vi "菜单-下载.vi"(8 "error in (no error)":errorcluster caption="错误输入（无错误）", 11 "程序响应 输入":refnum<class "程序响应.lvclass">) -> (0 "error out":errorcluster caption="错误输出", 3 "程序响应 输出":refnum<class "程序响应.lvclass">)   [LabVIEW 2020, in "程序响应.lvlib" / "程序响应.lvclass"]
uses:
  D:/SuperPython-master/ScintillaNET.dll
  ScintillaNET.dll
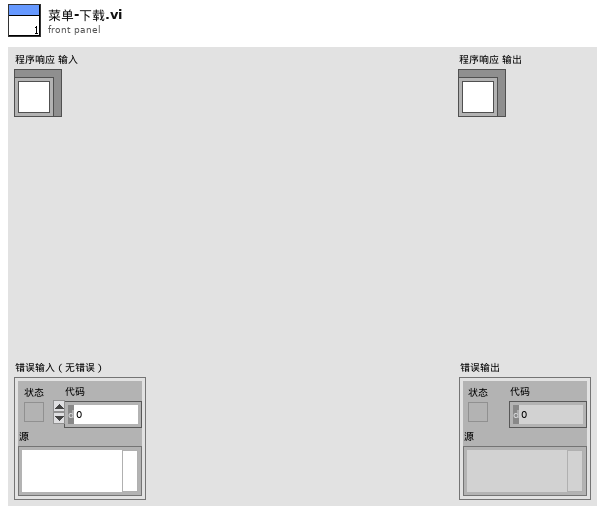
[diagram p1: front panel]
types:
  T1 = enum16{"open", "replace", "create", "open or create", "replace or create", "replace or create with confirmation"}
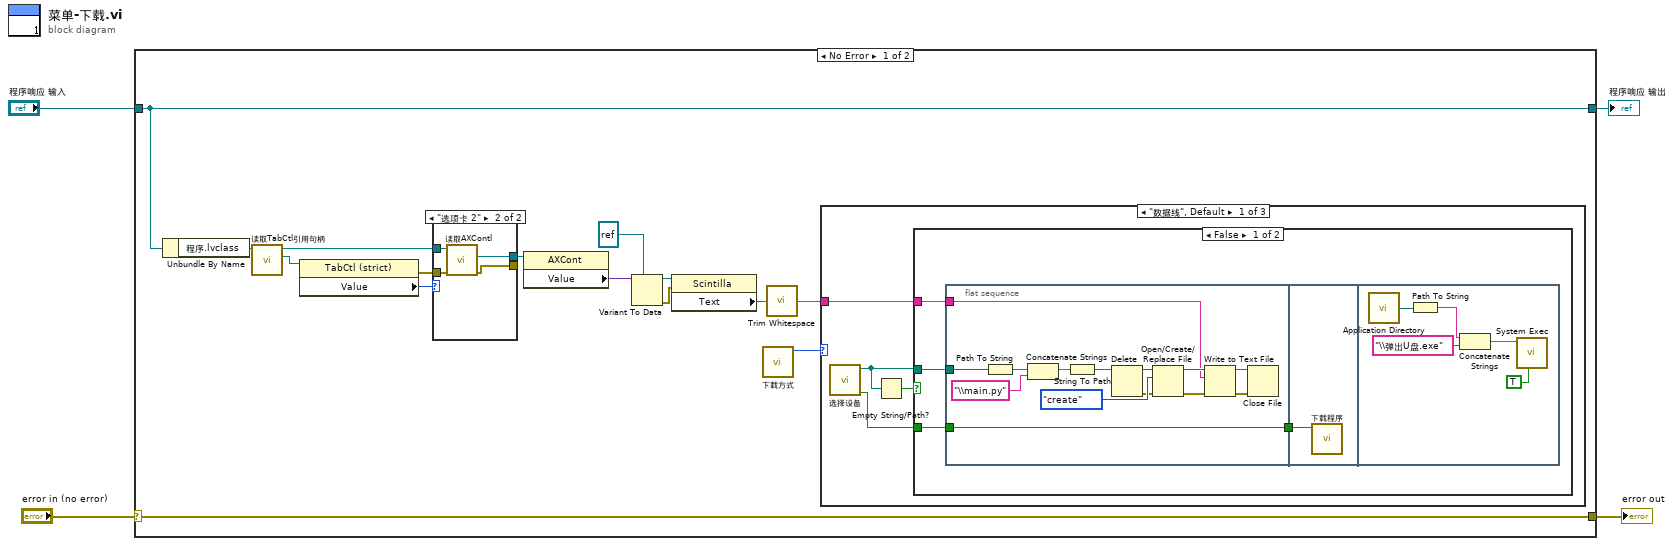
[diagram p0: block diagram]
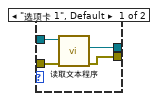
[diagram p2: hidden frame]
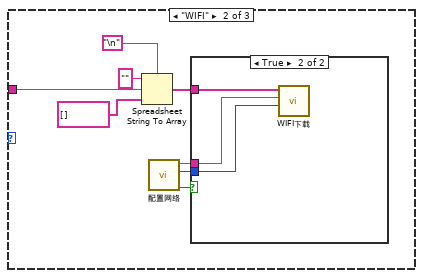
[diagram p4: hidden frame]
diagram:
  n1 = case shown="No Error" "error in (no error)" {
    selector: "error in (no error)" -> [w19 w68]
    tunnel: [w19 w68] -> w3
    tunnel: [w18 w67] -> w1
    tunnel: "程序响应 输入" -> [w18 w67]
    frame No Error {
      n2 = Unbundle By Name(w18) -> ("程序.lvclass"=w5:refnum<class "程序.lvclass">)
      n3 = call-dynamic "读取TabCtl引用句柄.vi"("程序输入"=w5) -> ("TabCtl引用句柄"=w10:refnum<vi>, "程序输出"=w7:refnum<class "程序.lvclass">)  [unwired: 8 in, 1 out]
      n4 = property class="TabCtl (strict)"(reference=w10) -> (error out=w8:errorcluster, "Value"=w9:enum32{"选项卡 1", "选项卡 2"})  [unwired: 1 in, 1 out]
      n5 = case shown="\"选项卡 2\"" w9 {
        tunnel: [w23 w24] -> w6
        tunnel: [w21 w25] -> _
        tunnel: w7 -> [w22 w27]
        tunnel: w8 -> [w20 w26]
        frame "选项卡 1", Default {
          n6 = call-dynamic "读取文本程序.vi"("error in (no error)"=w20, "程序输入"=w22) -> ("error out"=w21:errorcluster, "文本程序"=w23:refnum<vi>)  [unwired: 7 in, 1 out]
        }
        frame "选项卡 2" {
          n7 = call-dynamic "读取AXContl.vi"("error in (no error)"=w26, "程序输入"=w27) -> ("error out"=w25:errorcluster, "AXContl"=w24:refnum<vi>)  [unwired: 7 in, 1 out]
        }
      }
      n8 = property class="AXCont"(reference=w6) -> ("Value"=w12:variant)  [unwired: 1 in, 2 out]
      n9 = Variant To Data(type=refnum<k24> refnum ("文本编辑"), Variant=w12) -> (data=w13:refnum<k24>, error out=w14:errorcluster)  [unwired: 1 in]
      n10 = property class="Scintilla"(reference=w13, error in=w14) -> ("Text"=w11:string)  [unwired: 2 out]
      n11 = call "下载方式.vi"() -> ("下载方式"=w17:enum32{"数据线", "WIFI", "取消"})  [unwired: 11 in]
      n12 = call <vilib>:"Trim Whitespace.vi"("string"=w11) -> ("trimmed string"=w16:string)  [unwired: 1 in]
      n13 = case shown="\"数据线\", Default" w17 {
        tunnel: w16 -> [w31 w63 _]
        frame "数据线", Default {
          n14 = call "选择设备.vi"() -> ("boot?"=w28:bool, "路径"=w30:path)  [unwired: 10 in]
          n15 = Empty String/Path?(string/path=w30) -> (empty?=w29:bool)
          n16 = case shown="False" w29 {
            tunnel: w30 -> [w34 _]
            tunnel: w31 -> [w35 _]
            tunnel: w28 -> [w33 _]
            frame False {
              n17 = flat-sequence {
                tunnel: w35 -> [w44]
                tunnel: w34 -> [w43]
                tunnel: w33 -> [w36]
                tunnel: [w36] -> w32
                tunnel: w32 -> [w50]
                frame #0 {
                  n18 = Path To String(path=w43) -> (string=w40:string)
                  n19 = Concatenate Strings(w40, "\\main.py" ("名称或相对路径")) -> (w41:string)
                  n20 = String To Path(string=w41) -> (path=w39:path)
                  n21 = Delete(path (use dialog)=w39) -> (deleted path=w38:path, error out=w37:errorcluster)  [unwired: 4 in, 1 out]
                  n22 = Open/Create/Replace File(file path (use dialog)=w38, error in=w37, operation (0:open)=T1."create" ("操作(0:open)")) -> (refnum out=w49:refnum<file>, error out=w48:errorcluster)  [unwired: 3 in, 1 out]
                  n23 = Write to Text File(file (use dialog)=w49, text=w44, error in=w48) -> (refnum out=w47:refnum<file>, error out=w46:errorcluster)  [unwired: 1 in, 1 out]
                  n24 = Close File(refnum=w47, error in=w46) -> ()  [unwired: 2 out]
                }
                frame #1 {
                  n25 = call "下载程序.vi"("boot?"=w50) -> ()  [unwired: 11 in]
                }
                frame #2 {
                  n26 = call <vilib>:"Application Directory.vi"() -> ("Application Directory"=w55:path)
                  n27 = Path To String(path=w55) -> (string=w52:string)
                  n28 = Concatenate Strings(w52, "\\弹出U盘.exe" ("字符串")) -> (w53:string)
                  n29 = call <vilib>:"System Exec.vi"("run minimized? (F)"=TRUE, "command line"=w53) -> ()  [unwired: 6 in, 4 out]
                }
              }
            }
            frame True {
            }
          }
        }
        frame "WIFI" {
          n30 = Spreadsheet String To Array(delimiter (Tab)="\n", format string="" ("格式字符串"), spreadsheet string=w63, array type (2D Dbl)=string[] []) -> (array=w59:string[])
          n31 = call "配置网络.vi"() -> ("下载"=w56:bool, "端口号"=w57:u16, "IP"=w58:string)  [unwired: 9 in]
          n32 = case shown="True" w56 {
            tunnel: w59 -> [_ w66]
            tunnel: w58 -> [_ w65]
            tunnel: w57 -> [_ w64]
            frame False {
            }
            frame True {
              n33 = call "WIFI下载.vi"("远程端口"=w64, "地址"=w65, "程序"=w66) -> ()  [unwired: 9 in]
            }
          }
        }
        frame "取消" {
        }
      }
    }
    frame Error {
    }
  }
  "error out" <- w3
  "程序响应 输出" <- w1
